vi "Resize String To Text.vi"(4 "Min Height":u32=100, 5 "Max Size":T1={"Width"=800, "Height"=600}, 6 "Min Width":u32=200, 7 "Ratio (Width/Height)":dbl=1.61803399, 8 "error in (no error)":errorcluster, 11 "String Ref":refnum<vi>) -> (0 "error out":errorcluster, 3 "dup String Ref":refnum<vi>)   [LabVIEW 2013, in "Workspace MultiY Graph.lvlib" / "Alert Dialogs.lvlib"]
doc: "The string control is assumed fill a whole pane. The sting control is set to change size\nwith pane. If there are splitters in the window they \nare set to stick to left/right/top/bottom. There fore if we adjust the window it will adjust\nthe size of the control. If we just adjusted the control the window would not change."
uses:
  Alert Dialogs.lvlib
  <vilib>/Utility/miscctls.llb/LVBoundsTypeDef.ctl
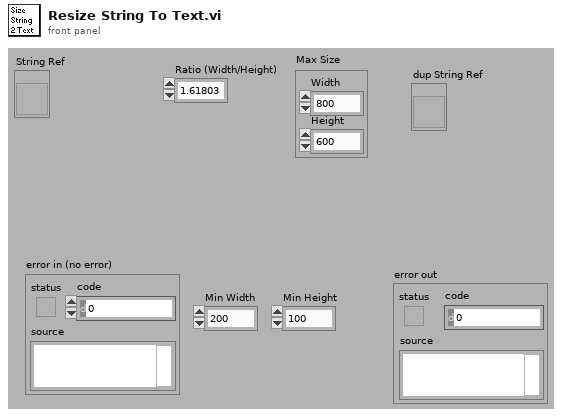
[diagram p1: front panel]
types:
  T1 = typedef "LVBoundsTypeDef.ctl" = cluster{"Width":u32, "Height":u32}
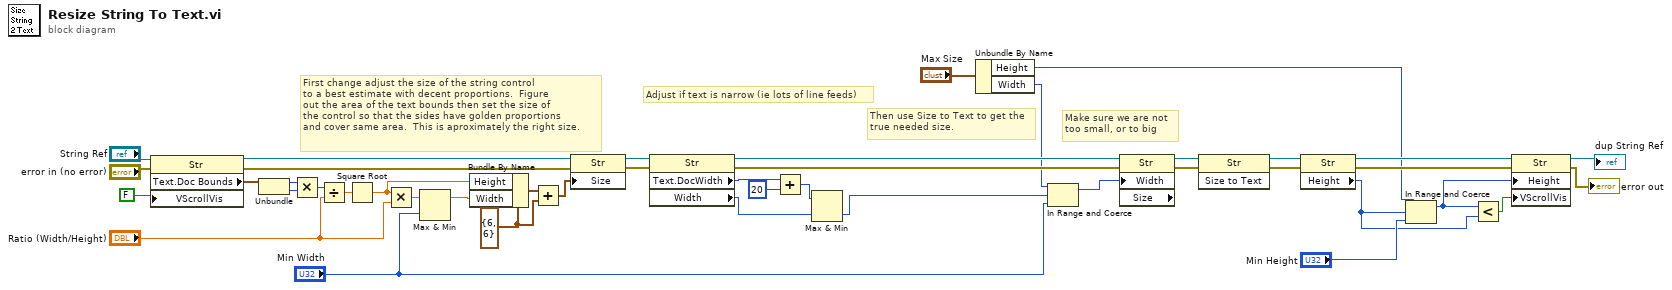
[diagram p0: block diagram]
diagram:
  w42 = T1 {"Width"=6, "Height"=6} ("Size")
  # "Adjust if text is narrow (ie lots of line feeds)"
  # "Make sure we are not too small, or to big"
  # "Then use Size to Text to get the\ntrue needed size."
  # "First change adjust the size of the string control\nto a best estimate with decent proportions.  Figure\nout the area of the text bounds then set the size of\nthe control so that the sides have golden proportions\nand cover same area.  This is aproximately the right size."
  n1 = property on="Property Node" class="Str"(reference="String Ref", error in="error in (no error)", "VScrollVis"=FALSE ("Vertical Scrollbar Visible")) -> (reference out=w37:refnum<vi>, error out=w38:errorcluster, "Text.Doc Bounds"=w39:T1)
  n2 = Unbundle(w39) -> ("Width"=w34:u32, "Height"=w35:u32)
  n3 = Multiply(x=w34, y=w35) -> (x*y=w31:u32)
  n4 = Divide(x=w31, y="Ratio (Width/Height)") -> (x/y=w30:dbl)
  n5 = Square Root(x=w30) -> (sqrt(x)=w40:dbl)
  n6 = Multiply(x=w40, y="Ratio (Width/Height)") -> (x*y=w29:dbl)
  n7 = Max & Min(x=w29, y="Min Width") -> (max(x,y)=w28:dbl)  [unwired: 1 out]
  n8 = Bundle By Name(cluster=w42, "Height"=w40, "Width"=w28) -> (w41:T1)
  n9 = Add(x=w41, y=w42) -> (x+y=w43:T1)
  n10 = property class="Str"(reference=w37, error in=w38, "Size"=w43) -> (reference out=w27:refnum<vi>, error out=w26:errorcluster)
  n11 = property on="Property Node" class="Str"(reference=w27, error in=w26) -> (reference out=w9:refnum<vi>, error out=w10:errorcluster, "Text.DocWidth"=w5:u32, "Width"=w3:u32)
  n12 = Add(x=w5, y=u32 20) -> (x+y=w2:u32)
  n13 = Max & Min(x=w2, y=w3) -> (min(x,y)=w1:u32)  [unwired: 1 out]
  n14 = Unbundle By Name("Max Size") -> ("Height"=w7:u32, "Width"=w6:u32)
  n15 = In Range and Coerce(upper limit=w6, x=w1, lower limit="Min Width") -> (coerced(x)=w24:u32)  [unwired: 1 out]
  n16 = property class="Str" props=["Width", "Size"](reference=w9, error in=w10, "Width"=w24) -> (reference out=w13:refnum<vi>, error out=w14:errorcluster)  [unwired: 1 out]
  n17 = invoke class="Str" method="Size to Text"(reference=w13, error in=w14) -> (reference out=w12:refnum<vi>, error out=w11:errorcluster)  [unwired: 1 in, 1 out]
  n18 = property class="Str"(reference=w12, error in=w11) -> (reference out=w19:refnum<vi>, error out=w20:errorcluster, "Height"=w22:u32)
  n19 = In Range and Coerce(upper limit=w7, x=w22, lower limit="Min Height") -> (coerced(x)=w21:u32)  [unwired: 1 out]
  n20 = Less?(x=w21, y=w22) -> (x < y?=w18:bool)
  n21 = property class="Str"(reference=w19, error in=w20, "Height"=w21, "VScrollVis"=w18) -> (reference out=→"dup String Ref":refnum<vi>, error out=→"error out":errorcluster)
